vi "Phasor Compute UC Tau Tick (g, s) & (dg, ds).vi"(8 "1/2 pi f":dbl[unit], 9 "Tick Length (0.01)":dbl=0.01, 10 "Tick Index":i32, 11 "tau_i":dbl[unit]) -> (0 "tau_i (ns)":dbl, 1 "label?":bool, 2 "Tick (dg, ds)":T1, 3 "Tick start (g, s)":T1, 4 "long tick?":bool)   [LabVIEW 2021, in "Phasor.lvlib"]
uses:
  Phasor.lvlib
  Phasor (g, s).ctl
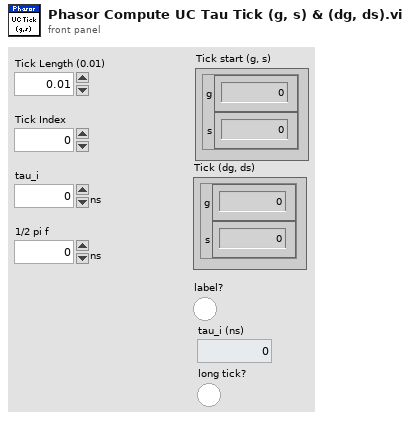
[diagram p1: front panel]
types:
  T1 = typedef "Phasor.lvlib/Phasor (g, s).ctl" = cluster{"g":dbl, "s":dbl}
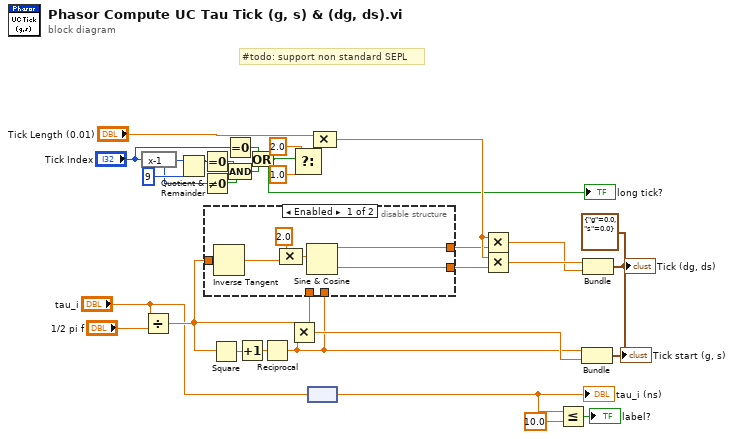
[diagram p0: block diagram]
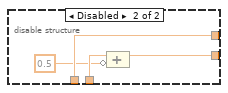
[diagram p2: hidden frame]
diagram:
  w1 = T1 {"g"=0.0, "s"=0.0} ("Tick center (g, s)")
  # "#todo: support non standard SEPL"
  n1 = expression code="x-1"("Tick Index") -> (w28:i32)
  n2 = Divide(x="tau_i", y="1/2 pi f") -> (x/y=w16:dbl)
  n3 = Quotient & Remainder(x=w28, y=9 ("# Decades")) -> (x-y*floor(x/y)=w21:i32)  [unwired: 1 out]
  n4 = Equal To 0?(x=w21) -> (x = 0?=w27:bool)
  n5 = Not Equal To 0?(x=w28) -> (x != 0?=w30:bool)
  n6 = Square(x=w16) -> (x^2=w14:dbl)
  n7 = Equal To 0?(x="Tick Index") -> (x = 0?=w26:bool)
  n8 = Compound Arithmetic op=AND(w27, w30) -> (w29:bool)
  n9 = Increment(x=w14) -> (x+1=w15:dbl)
  n10 = Or(x=w26, y=w29) -> (x .or. y?=w4:bool)
  "long tick?" <- w4
  n11 = Reciprocal(x=w15) -> (1/x=w2:dbl)
  n12 = Multiply(x=w16, y=w2) -> (x*y=w3:dbl)
  n13 = disable-structure shown="Enabled" {
    disable-tunnel: [w35 w39] -> w18
    disable-tunnel: [w34 w41] -> w17
    disable-tunnel: w16 -> [w33 _]
    disable-tunnel: w3 -> [_ w41]
    disable-tunnel: w2 -> [_ w40]
    frame Enabled {
      n14 = Inverse Tangent(1:w33) -> (0:w32:dbl)
      n15 = Compound Arithmetic op=MULTIPLY(2.0 ("value"), w32) -> (w36:dbl)
      n16 = Sine & Cosine(0:w36) -> (1:w34:dbl, 2:w35:dbl)
    }
    frame Disabled {
      n17 = Compound Arithmetic op=ADD(w40, invert 0.5 ("value")) -> (w39:dbl)
    }
  }
  n18 = Select(t=2.0 ("value"), s=w4, f=1.0) -> (s? t:f=w24:dbl)
  n19 = node("tau_i") -> (w7:dbl)
  "tau_i (ns)" <- w7
  n20 = Compound Arithmetic op=MULTIPLY("Tick Length (0.01)", w24) -> (w20:dbl)
  n21 = Multiply(x=w20, y=w17) -> (x*y=w11:dbl)
  n22 = Multiply(x=w20, y=w18) -> (x*y=w12:dbl)
  n23 = Less Or Equal?(x=w7, y=10.0) -> (x <= y?=→"label?":bool)
  n24 = Bundle(cluster=w1, "g"=w2, "s"=w3) -> (→"Tick start (g, s)":T1)
  n25 = Bundle(cluster=w1, "g"=w12, "s"=w11) -> (→"Tick (dg, ds)":T1)
